vi "Counter Synch-Analog Task 2012 NIVerified.vi"() -> ()   [LabVIEW 2012]
doc: "The VI creates a dummy Analog Input task, and use the AI Sample Clock as the clock source for both counters."
uses:
  <vilib>/Utility/error.llb/DialogType.ctl
  <vilib>/DAQmx/configure/timing.llb/DAQmx Timing (Sample Clock).vi
  <vilib>/DAQmx/create/channels.llb/DAQmx Create Channel (CI-Count Edges).vi
  <vilib>/DAQmx/create/channels.llb/DAQmx Create Channel (AI-Voltage-Basic).vi
  <vilib>/DAQmx/read.llb/DAQmx Read (Counter 1D DBL 1Chan NSamp).vi
panel:
  out "data 2":dbl[](array[numeric]) caption="Counter 1 Data" format="%0.2f"
  out "data":dbl[](array[numeric]) caption="Counter 0 Data" format="%0.2f"
  in  "Sample Clock Source":tag="/Dev1/ai/SampleClock"
  in  "rate":dbl=1000.0 format="%0.2f"
  in  "Physical Channel 0":tag="Dev1/ai0"
  in  "active edge 2":i32(ring)=10280 caption="active edge" items=["Rising"=10280, "Falling"=10171]
  in  "active edge":i32(ring)=10280 items=["Rising"=10280, "Falling"=10171]
  in  "Physical Channel 2":tag="Dev1/ctr1"
  in  "Physical Channel 1":tag="Dev1/ctr0"
  in  "stop":bool
  # "Overview:The VI creates a dummy Analog Input task, and use the AI Sample Clock as the clock source for both counters.\nRequirements:\n•\tLabVIEW 2012 (or compatible)\n•\tNI DAQmx 12.0 (or compatible)\nInstructions:\n1.Select the channel of Analog Channel Properties control, Counter 0 Channel Properties control and Counter 1 Channel Properties control .\n2.Run the VI"
  # "Analog Channel Properties"
  # "Counter 0 Channel Properties"
  # "Counter 1 Channel Properties"
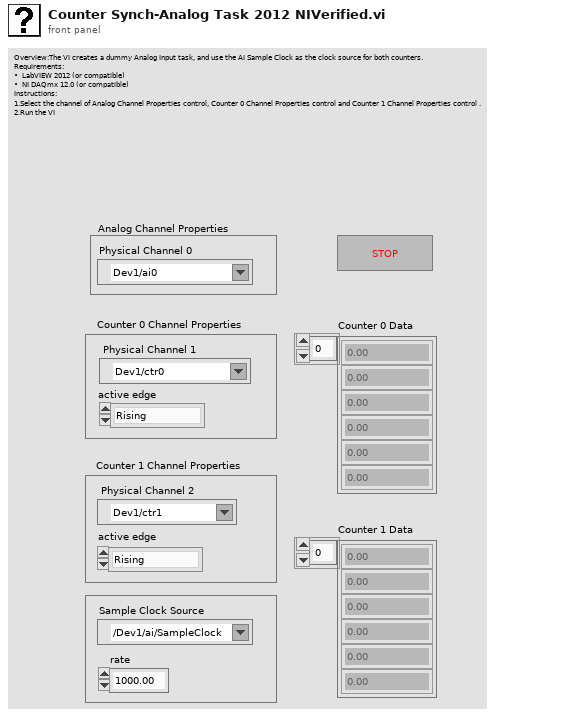
[diagram p1: front panel]
types:
  T1 = typedef "DialogType.ctl" = u16
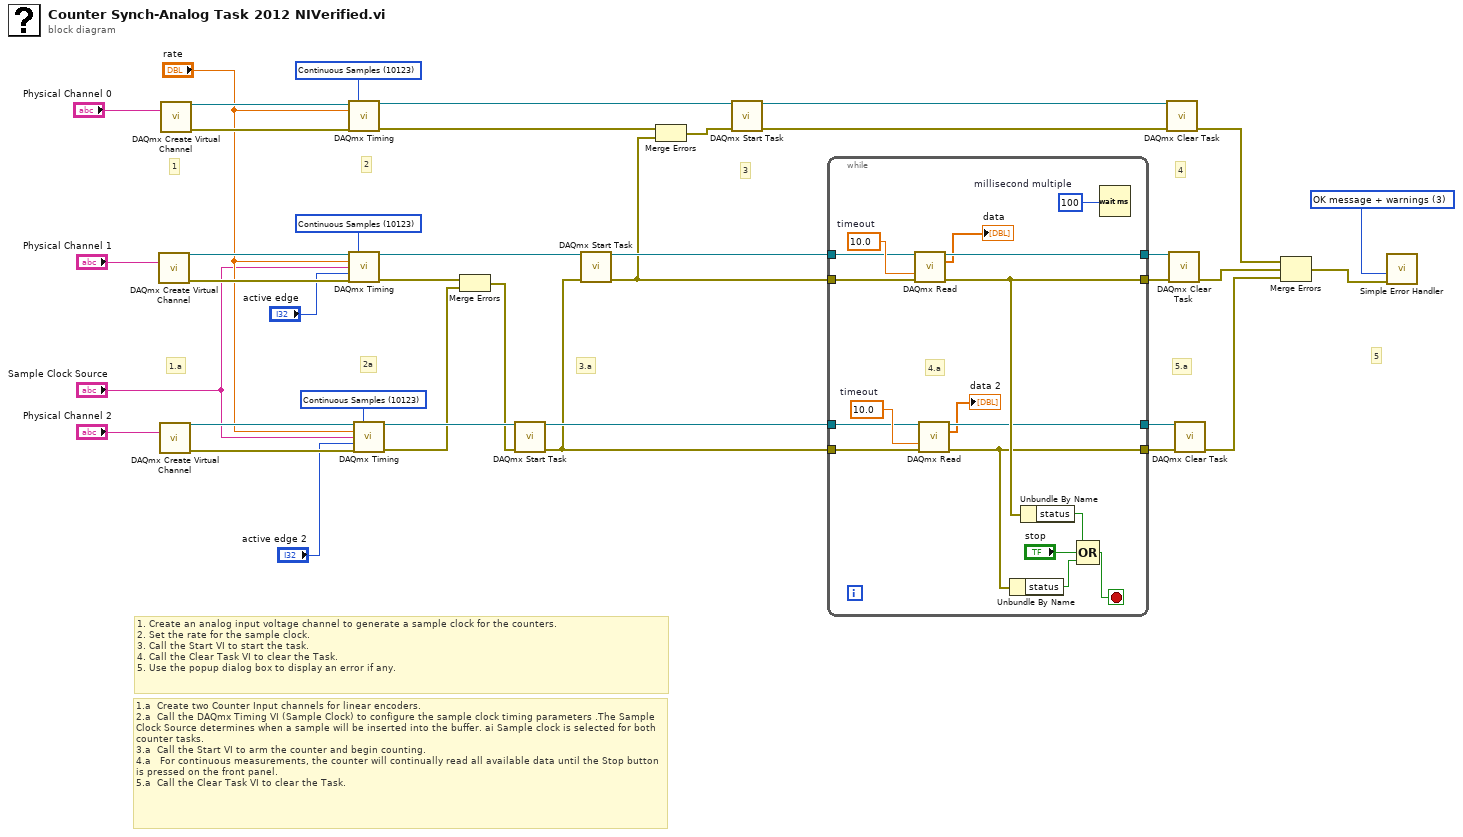
[diagram p0: block diagram]
diagram:
  w4 = 10123 items=["Finite Samples"=10178, "Continuous Samples"=10123, "Hardware Timed Single Point"=12522] ("sample mode")
  w5 = 10123 items=["Finite Samples"=10178, "Continuous Samples"=10123, "Hardware Timed Single Point"=12522] ("sample mode")
  w6 = 10123 items=["Finite Samples"=10178, "Continuous Samples"=10123, "Hardware Timed Single Point"=12522] ("sample mode")
  w21 = T1 3 items=["no dialog", "OK message", "continue or stop message", "OK message + warnings", "continue/stop + warnings"] ("type of dialog (OK msg:1)")
  # "1. Create an analog input voltage channel to generate a sample clock for the counters.\n2. Set the rate for the sample clock.\n3. Call the Start VI to start the task.\n4. Call the Clear Task VI to clear the Task.\n5. Use the popup dialog box to display an error if any."
  # "5"
  # "1.a  Create two Counter Input channels for linear encoders. \n2.a  Call the DAQmx Timing VI (Sample Clock) to configure the sample clock timing parameters .The Sample Clock Source determines when a sample will be inserted into the buffer. ai Sample clock is selected for both counter tasks.\n3.a  Call the Start VI to arm the counter and begin counting.\n4.a   For continuous measurements, the counter will continually read all available data until the Stop button is pressed on the front panel.\n5.a  Call the Clear Task VI to clear the Task."
  # "5.a"
  # "3.a"
  # "2a"
  # "1.a"
  # "4"
  # "3"
  # "2"
  # "1"
  n1 = call-poly <vilib>:"DAQmx Create Virtual Channel.vi"("counter"="Physical Channel 1") -> ("task out"=w37:refnum<k21>, "error out"=w36:errorcluster)  [unwired: 6 in, 7 out]
  n2 = call-poly <vilib>:"DAQmx Create Virtual Channel.vi"("counter"="Physical Channel 2") -> ("task out"=w32:refnum<k21>, "error out"=w33:errorcluster)  [unwired: 6 in, 7 out]
  n3 = call-poly <vilib>:"DAQmx Create Virtual Channel.vi"("physical channels"="Physical Channel 0") -> ("task out"=w39:refnum<k21>, "error out"=w38:errorcluster)  [unwired: 8 in, 5 out]
  n4 = call-poly <vilib>:"DAQmx Timing.vi"("task/channels in"=w39, "sample mode"=w6, "rate"="rate", "error in"=w38) -> ("task out"=w29:refnum<k21>, "error out"=w25:errorcluster)  [unwired: 3 in, 7 out]
  n5 = call-poly <vilib>:"DAQmx Timing.vi"("task/channels in"=w37, "sample mode"=w4, "rate"="rate", "source"="Sample Clock Source", "active edge"="active edge", "error in"=w36) -> ("task out"=w31:refnum<k21>, "error out"=w28:errorcluster)  [unwired: 1 in, 7 out]
  n6 = call-poly <vilib>:"DAQmx Timing.vi"("task/channels in"=w32, "sample mode"=w5, "rate"="rate", "source"="Sample Clock Source", "active edge"="active edge 2", "error in"=w33) -> ("task out"=w30:refnum<k21>, "error out"=w26:errorcluster)  [unwired: 1 in, 7 out]
  n7 = Merge Errors(w28, w26) -> (w27:errorcluster)
  n8 = call <vilib>:"DAQmx Start Task.vi"("task/channels in"=w30, "error in"=w27) -> ("task out"=w16:refnum<k21>, "error out"=w15:errorcluster)  [unwired: 12 out]
  n9 = call <vilib>:"DAQmx Start Task.vi"("task/channels in"=w31, "error in"=w15) -> ("task out"=w18:refnum<k21>, "error out"=w17:errorcluster)  [unwired: 12 out]
  n10 = Merge Errors(w25, w17) -> (w24:errorcluster)
  n11 = call <vilib>:"DAQmx Start Task.vi"("task/channels in"=w29, "error in"=w24) -> ("task out"=w2:refnum<k21>, "error out"=w1:errorcluster)  [unwired: 12 out]
  n12 = while {
    tunnel: w17 -> [w56]
    tunnel: [w50] -> w23
    tunnel: [w52] -> w22
    tunnel: w16 -> [w48]
    tunnel: w15 -> [w47]
    tunnel: [w46] -> w20
    tunnel: [w43] -> w19
    tunnel: w18 -> [w45]
    stop <- w55 stop-if-true
    w49 = 10.0  # timeout
    w40 = u32 100  # millisecond multiple
    w51 = 10.0  # timeout
    # "4.a"
    n13 = call-poly <vilib>:"DAQmx Read.vi"("task/channels in"=w45, "timeout"=w51, "error in"=w56) -> ("task out"=w52:refnum<k21>, "data"=→"data":dbl[], "error out"=w50:errorcluster)  [unwired: 1 in, 9 out]
    n14 = call-poly <vilib>:"DAQmx Read.vi"("task/channels in"=w48, "timeout"=w49, "error in"=w47) -> ("task out"=w46:refnum<k21>, "data"=→"data 2":dbl[], "error out"=w43:errorcluster)  [unwired: 1 in, 9 out]
    n15 = Unbundle By Name(w43) -> ("status"=w44:bool)
    n16 = Unbundle By Name(w50) -> ("status"=w53:bool)
    n17 = Compound Arithmetic op=OR(w53, "stop", w44) -> (w55:bool)
    n18 = Wait (ms)(milliseconds to wait=w40) -> ()  [unwired: 1 out]
  }
  n19 = call <vilib>:"DAQmx Clear Task.vi"("task in"=w2, "error in"=w1) -> ("error out"=w13:errorcluster)  [unwired: 13 out]
  n20 = call <vilib>:"DAQmx Clear Task.vi"("task in"=w22, "error in"=w23) -> ("error out"=w14:errorcluster)  [unwired: 13 out]
  n21 = call <vilib>:"DAQmx Clear Task.vi"("task in"=w20, "error in"=w19) -> ("error out"=w12:errorcluster)  [unwired: 13 out]
  n22 = Merge Errors(w13, w14, w12) -> (w11:errorcluster)
  n23 = call <vilib>:"Simple Error Handler.vi"("type of dialog (OK msg:1)"=w21, "error in (no error)"=w11) -> ()  [unwired: 8 out]
